vi "Close.vi"(8 "error in (no error)":errorcluster, 11 "State in":T1={"State"=enum."Idle", "Start Time"=timestamp(0 s since 1904-01-01), "Configuration"={"Cycle Period"=0.0, "Ismatech"={"VISA resource name"="", "Simulated?"=FALSE, "Pump Number"=1.0, "Reverse?"=FALSE}, "Masterflex"={"VISA resource name"="", "Simulated?"=FALSE, "Pump Number"=1.0, "Reverse?"=FALSE}, "Manual Entry"=0.0, "VICI Settings"={"VISA resource name"="", "Simulated?"=FALSE, "Pump Letter"="", "Reverse?"=FALSE}, "Output Device"=enum."Ismatec ISM 831C", "Tacmina Settings"={"Analog DAQ Task"="", "Digital DAQ Task"=""}, "KNF SIMDOS Settings"={"VISA resource name"="", "Simulated?"=TRUE}, "ASIA Pump C"={"ASIA Pump #"=0, "channel"=0, "Simulated"=FALSE}, "FLOM Settings"={"VISA resource name"="", "Simulated?"=TRUE, "Pump Number"=0.0}, "Pump Calibration File"=path "", "Calibration Slope"=0.0, "Calibration Y Intercept"=0.0, "Pump Cal Enum"=0, "SSI PR Settings"={"VISA resource name"="", "Simulated?"=FALSE}}, "Current Time"=timestamp(0 s since 1904-01-01), "First Iteration"=FALSE, "Data"={"Pump Speed"=0.0, "Pump Pressure"=0.0, "Pump Flow"=0.0}, "Process Name"="", "Pump On?"=enum."Off", "Output Error"=FALSE, "Log Started"=FALSE, "Overpressure Alarming"=FALSE} {"Configuration"."ASIA Pump C"."channel" min=0 max=1 step=1; "Configuration"."Masterflex"."Pump Number" min=1.0 max=20.0 step=1.0; "Configuration"."Ismatech"."Pump Number" min=1.0 max=20.0 step=1.0}) -> (0 "error out":errorcluster, 3 "State out":T1={"State"=enum."Idle", "Start Time"=timestamp(0 s since 1904-01-01), "Configuration"={"Cycle Period"=0.0, "Ismatech"={"VISA resource name"="", "Simulated?"=FALSE, "Pump Number"=1.0, "Reverse?"=FALSE}, "Masterflex"={"VISA resource name"="", "Simulated?"=FALSE, "Pump Number"=1.0, "Reverse?"=FALSE}, "Manual Entry"=0.0, "VICI Settings"={"VISA resource name"="", "Simulated?"=FALSE, "Pump Letter"="", "Reverse?"=FALSE}, "Output Device"=enum."Ismatec ISM 831C", "Tacmina Settings"={"Analog DAQ Task"="", "Digital DAQ Task"=""}, "KNF SIMDOS Settings"={"VISA resource name"="", "Simulated?"=TRUE}, "ASIA Pump C"={"ASIA Pump #"=0, "channel"=0, "Simulated"=FALSE}, "FLOM Settings"={"VISA resource name"="", "Simulated?"=TRUE, "Pump Number"=0.0}, "Pump Calibration File"=path "", "Calibration Slope"=0.0, "Calibration Y Intercept"=0.0, "Pump Cal Enum"=0, "SSI PR Settings"={"VISA resource name"="", "Simulated?"=FALSE}}, "Current Time"=timestamp(0 s since 1904-01-01), "First Iteration"=FALSE, "Data"={"Pump Speed"=0.0, "Pump Pressure"=0.0, "Pump Flow"=0.0}, "Process Name"="", "Pump On?"=enum."Off", "Output Error"=FALSE, "Log Started"=FALSE, "Overpressure Alarming"=FALSE} {"Configuration"."ASIA Pump C"."channel" min=0 max=1 step=1; "Configuration"."Masterflex"."Pump Number" min=1.0 max=20.0 step=1.0; "Configuration"."Ismatech"."Pump Number" min=1.0 max=20.0 step=1.0})   [LabVIEW 2018, in "Pump Module.lvlib" / "Pump Module Engine.lvlib"]
uses:
  Pump Module Engine.lvlib
  State Cluster.ctl
  State Enum.ctl
  Pump Module Settings Cluster.ctl
  Ismatec ISM 831C/Controls/Ismatech Settings Cluster.ctl
  Masterflex 7550-30/Controls/Settings Cluster.ctl
  VICI M50 Party Mode/Settings Cluster.ctl
  Measure Instrument/PID 2 Output Enum.ctl
  Tacmina QI/Tacmina QI DAQ Setting.ctl
  KNF Pump/Settings Cluster plus SIMDOS.ctl
  ASIA Pump/Pump Settings.ctl
  FLOM Pump/Settings Cluster.ctl
  SSI PR Class/SSI PR Settings Cluster.ctl
  Tag VIs/Tag FGV Operation Enum.ctl
  Masterflex 7550-30/Masterflex 7550-30.lvlib
  Ismatec ISM 831C/Ismatec ISM 831C.lvlib
  Tacmina QI/Tacmina QI.lvlib
  VICI M50 Party Mode/VICI M6 M50 Party Mode.lvlib
  ASIA Pump.lvlib
  KNF Pump/KNF SIMDOS.lvlib
  FLOM Pump/FLOM Pump.lvlib
  SSI PR Class/SSI PR Pump.lvlib
  Shared Variables/Dynamic Shared Variables.lvlib
  Pump Module.lvlib
panel:
  # "Output Instruments"
  # "Output Instruments"
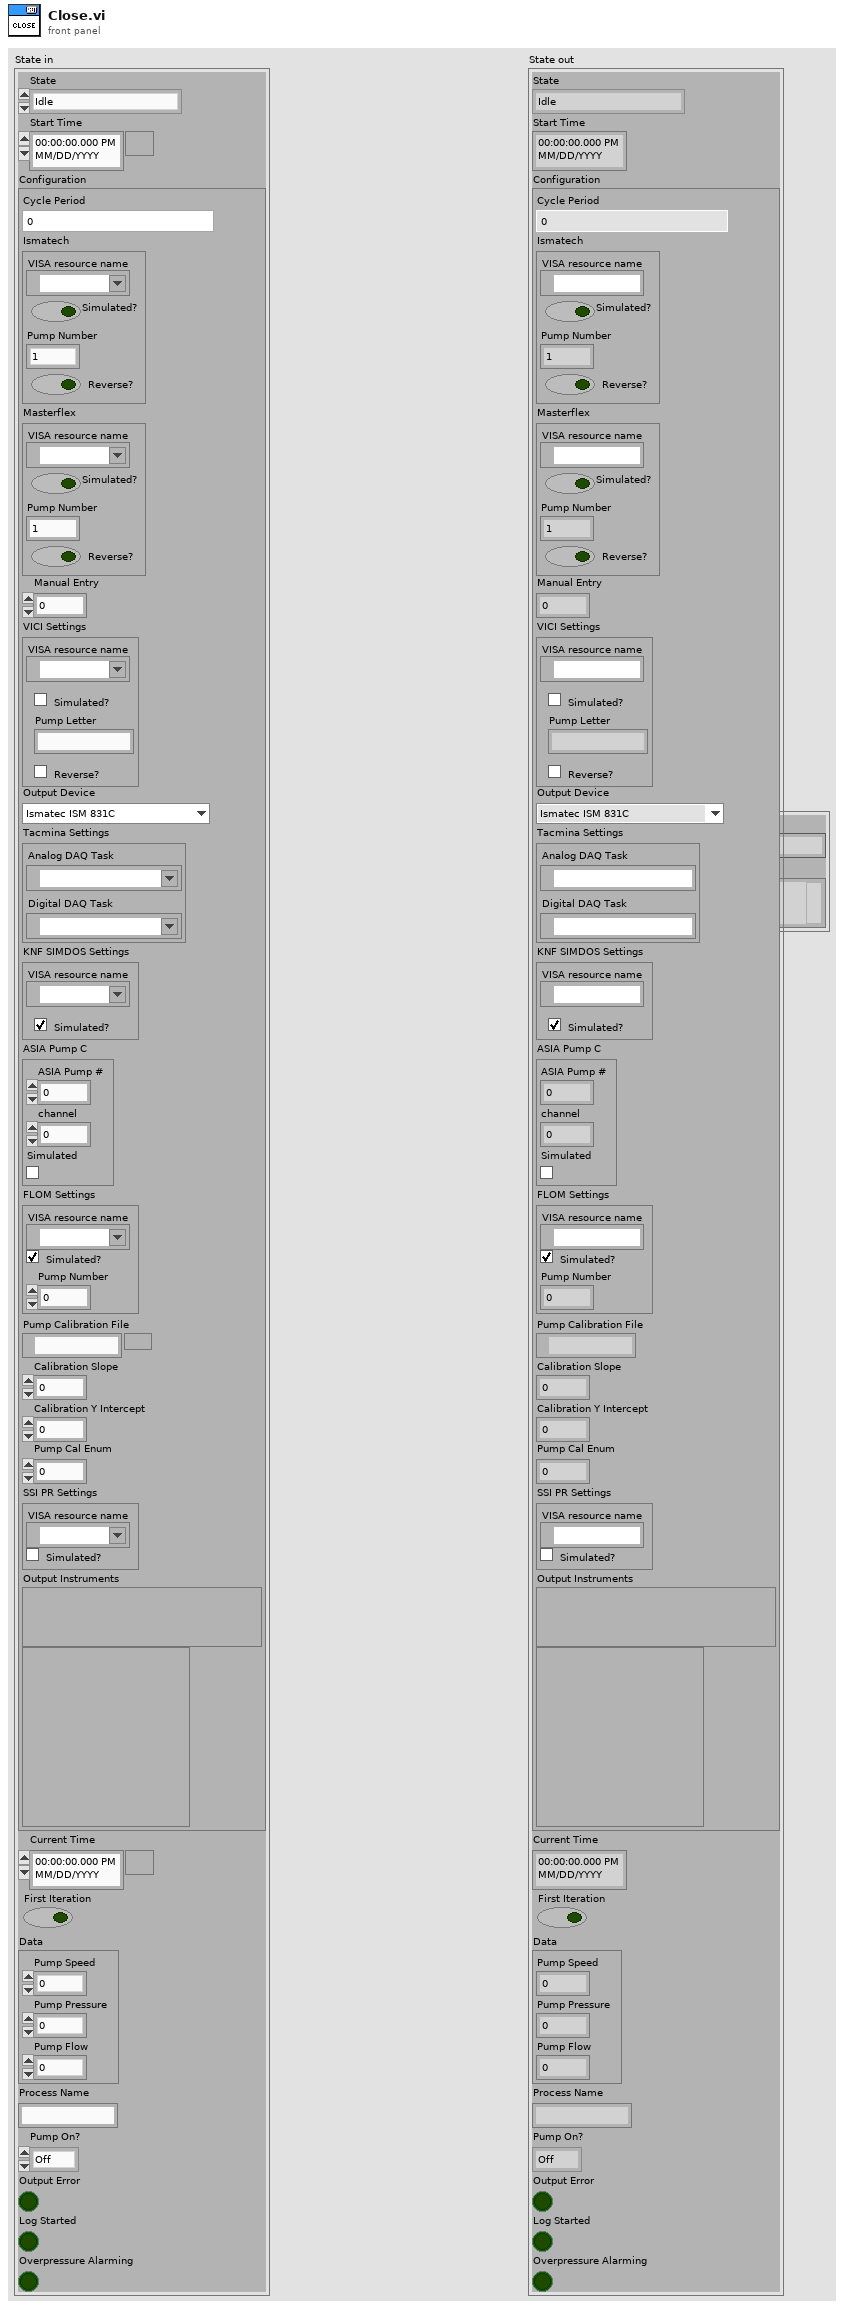
[diagram p1: front panel]
types:
  T1 = typedef "Pump Module.lvlib/Pump Module Engine.lvlib/State Cluster.ctl" = cluster{"State":T2, "Start Time":timestamp, "Configuration":T3, "Current Time":timestamp, "First Iteration":bool, "Data":cluster{"Pump Speed":dbl, "Pump Pressure":dbl, "Pump Flow":dbl}, "Process Name":string, "Pump On?":enum16{"Off", "On", "Not Initialized"}, "Output Error":bool, "Log Started":bool, "Overpressure Alarming":bool}
  T2 = typedef "Pump Module.lvlib/Pump Module Engine.lvlib/State Enum.ctl" = enum16{"Measuring", "Idle", "Paused"}
  T3 = typedef "Pump Module.lvlib/Pump Module Settings Cluster.ctl" = cluster{"Cycle Period":dbl, "Ismatech":T4, "Masterflex":T5, "Manual Entry":dbl, "VICI Settings":T6, "Output Device":T7, "Tacmina Settings":T8, "KNF SIMDOS Settings":T9, "ASIA Pump C":T10, "FLOM Settings":T11, "Pump Calibration File":path, "Calibration Slope":dbl, "Calibration Y Intercept":dbl, "Pump Cal Enum":u16, "SSI PR Settings":T12}
  T4 = typedef "Ismatec ISM 831C.lvlib/Ismatech Settings Cluster.ctl" = cluster{"VISA resource name":refnum<visa-resource-name>, "Simulated?":bool, "Pump Number":dbl, "Reverse?":bool}
  T5 = typedef "Masterflex 7550-30.lvlib/Settings Cluster.ctl" = cluster{"VISA resource name":refnum<visa-resource-name>, "Simulated?":bool, "Pump Number":dbl, "Reverse?":bool}
  T6 = typedef "VICI M6 M50 Party Mode.lvlib/Settings Cluster.ctl" = cluster{"VISA resource name":refnum<visa-resource-name>, "Simulated?":bool, "Pump Letter":string, "Reverse?":bool}
  T7 = typedef "PID 2 Output Enum.ctl" = enum16{"Default", "Ismatec ISM 831C", "Masterflex 7550-30", "VICI", "Tacmina QI", "KNF SIMDOS", "ASIA Type C", "FLOM UI-22-11", "SSI PR"}
  T8 = typedef "Tacmina QI.lvlib/Tacmina QI DAQ Setting.ctl" = cluster{"Analog DAQ Task":refnum<k21>, "Digital DAQ Task":refnum<k21>}
  T9 = typedef "KNF SIMDOS.lvlib/Settings Cluster plus SIMDOS.ctl" = cluster{"VISA resource name":refnum<visa-resource-name>, "Simulated?":bool}
  T10 = typedef "ASIA Pump.lvlib/Pump Settings.ctl" = cluster{"ASIA Pump #":i32, "channel":i32, "Simulated":bool}
  T11 = typedef "FLOM Pump.lvlib/Settings Cluster.ctl" = cluster{"VISA resource name":refnum<visa-resource-name>, "Simulated?":bool, "Pump Number":dbl}
  T12 = typedef "SSI PR Pump.lvlib/SSI PR Settings Cluster.ctl" = cluster{"VISA resource name":refnum<visa-resource-name>, "Simulated?":bool}
  T13 = typedef "Pump Module.lvlib/Pump Module Tag Names Cluster.ctl" = cluster{"Pump Speed":string, "Pump Flow":string, "Pump Pressure":string, "Output Device Tag":string, "Overpressure Tag":string}
  T14 = typedef "Tag FGV Operation Enum.ctl" = enum16{"Init", "Set Notification Queue", "Create Tag", "Commit", "Write Tag (Numeric)", "Write Tag (Boolean)", "Read All Tags", "Read One Tag", "Delete Tag Category", "Set Alarm Parameters (Numeric)", "Set Alarm Parameters (Boolean)", "Enable All Alarms", "Disable All Alarms", "Delete All Tags", "Read Alarms", "Ack Alarm", "Read Alarm Parameters (Numeric)", "Read Alarm Parameters (Boolean)"}
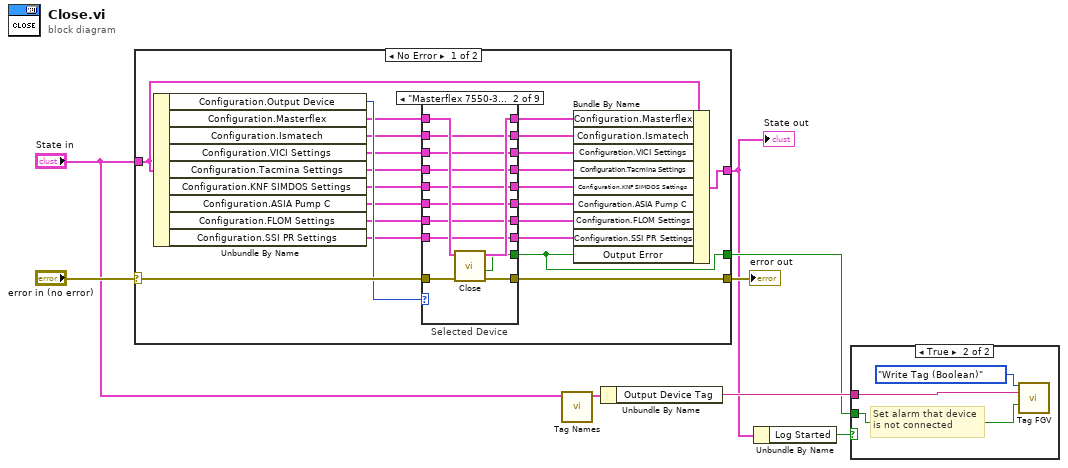
[diagram p0: block diagram]
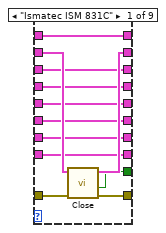
[diagram p3: hidden frame]
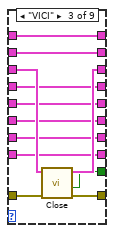
[diagram p4: hidden frame]
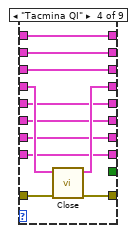
[diagram p5: hidden frame]
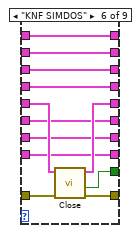
[diagram p7: hidden frame]
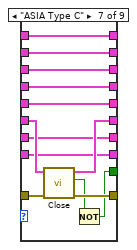
[diagram p8: hidden frame]
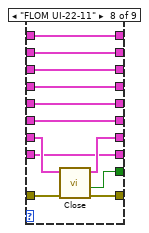
[diagram p9: hidden frame]
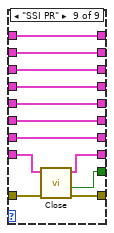
[diagram p10: hidden frame]
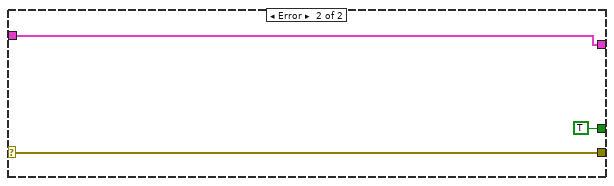
[diagram p11: hidden frame]
diagram:
  n1 = case shown="No Error" "error in (no error)" {
    selector: "error in (no error)" -> [w25 w138]
    tunnel: [w28 w138] -> w7
    tunnel: "State in" -> [w20 w137]
    tunnel: [w30 w137] -> w2
    tunnel: [w9 TRUE ("Connection Error")] -> w3
    frame No Error {
      n2 = Unbundle By Name(w20) -> ("Configuration.Output Device"=w19:T7, "Configuration.Masterflex"=w18:T5, "Configuration.Ismatech"=w17:T4, "Configuration.VICI Settings"=w16:T6, "Configuration.Tacmina Settings"=w15:T8, "Configuration.KNF SIMDOS Settings"=w14:T9, "Configuration.ASIA Pump C"=w13:T10, "Configuration.FLOM Settings"=w12:T11, "Configuration.SSI PR Settings"=w11:T12)
      n3 = case "Selected Device" shown="\"Masterflex 7550-30\"" w19 {
        tunnel: w18 -> [w38 w54 w61 w74 w86 w94 w109 w123 w135]
        tunnel: [w38 w53 w61 w74 w86 w94 w109 w123 w135] -> w29
        tunnel: w17 -> [w40 w51 w62 w75 w82 w93 w108 w122 w134]
        tunnel: [w42 w52 w64 w76 w85 w97 w110 w116 w127] -> w28
        tunnel: w25 -> [w41 w50 w65 w77 w85 w98 w111 w117 w128]
        tunnel: [w39 w51 w62 w75 w82 w93 w108 w122 w134] -> w27
        tunnel: w16 -> [w37 w49 w66 w72 w84 w92 w107 w121 w133]
        tunnel: [w37 w49 w63 w72 w84 w92 w107 w121 w133] -> w26
        tunnel: w15 -> [w36 w48 w60 w71 w83 w91 w106 w120 w132]
        tunnel: [w36 w48 w60 w73 w83 w91 w106 w120 w132] -> w24
        tunnel: w14 -> [w35 w47 w58 w70 w80 w96 w105 w119 w131]
        tunnel: [w35 w47 w58 w70 w80 w95 w105 w119 w131] -> w23
        tunnel: [w34 w46 w59 w69 w81 w90 w103 w118 w130] -> w22
        tunnel: w13 -> [w34 w46 w59 w69 w81 w90 w104 w118 w130]
        tunnel: w12 -> [w33 w45 w57 w68 w79 w89 w102 w115 w129]
        tunnel: [w33 w45 w57 w68 w79 w89 w102 w114 w129] -> w21
        tunnel: w11 -> [w32 w44 w56 w67 w78 w88 w101 w113 w126]
        tunnel: [w32 w44 w56 w67 w78 w88 w101 w113 w125] -> w10
        tunnel: [w31 w43 w55 _ _ w87 w99 w112 w124] -> w9
        frame "Ismatec ISM 831C" {
          n4 = call "Close.vi"("error in (no error)"=w41, "Ismatech Settings"=w40) -> ("error out"=w42:errorcluster, "Connection Error"=w31:bool, "Ismatech Settings"=w39:T4)  [unwired: 7 in]
        }
        frame "Masterflex 7550-30" {
          n5 = call "Close.vi"("error in (no error)"=w50, "Masterflex Settings in"=w54) -> ("error out"=w52:errorcluster, "Connection Error"=w43:bool, "Masterflex Settings out"=w53:T5)  [unwired: 7 in]
        }
        frame "VICI" {
          n6 = call "Close.vi"("error in (no error)"=w65, "VICI Settings"=w66) -> ("error out"=w64:errorcluster, "Connection Error"=w55:bool, "VICI Settings"=w63:T6)  [unwired: 7 in]
        }
        frame "Tacmina QI" {
          n7 = call "Close.vi"("error in"=w77, "Tacmina Settings in"=w71) -> ("error out"=w76:errorcluster, "Tacmina Settings out"=w73:T8)  [unwired: 8 in]
        }
        frame "Default", Default {
        }
        frame "KNF SIMDOS" {
          n8 = call "Close.vi"("error in (no error)"=w98, "KNF Settings"=w96) -> ("error out"=w97:errorcluster, "Connection Error"=w87:bool, "KNF Settings"=w95:T9)  [unwired: 7 in]
        }
        frame "ASIA Type C" {
          n9 = call "Close.vi"("error in (no error)"=w111, "ASIA Pump C"=w104) -> ("error out"=w110:errorcluster, "Task Completed"=w100:bool, "ASIA Pump C"=w103:T10)  [unwired: 7 in]
          n10 = Not(x=w100) -> (.not. x?=w99:bool)
        }
        frame "FLOM UI-22-11" {
          n11 = call "Close.vi"("error in (no error)"=w117, "FLOM Settings in"=w115) -> ("error out"=w116:errorcluster, "Connection Error"=w112:bool, "FLOM Settings out"=w114:T11)  [unwired: 7 in]
        }
        frame "SSI PR" {
          n12 = call "Close.vi"("error in (no error)"=w128, "SSI PR Settings In"=w126) -> ("error out"=w127:errorcluster, "Connection Error"=w124:bool, "SSI PR Settings Out"=w125:T12)  [unwired: 7 in]
        }
      }
      n13 = Bundle By Name(cluster=w20, "Configuration.Masterflex"=w29, "Configuration.Ismatech"=w27, "Configuration.VICI Settings"=w26, "Configuration.Tacmina Settings"=w24, "Configuration.KNF SIMDOS Settings"=w23, "Configuration.ASIA Pump C"=w22, "Configuration.FLOM Settings"=w21, "Configuration.SSI PR Settings"=w10, "Output Error"=w9) -> (w30:T1)
    }
    frame Error {
    }
  }
  "error out" <- w7
  "State out" <- w2
  n14 = call "Tag Names.vi"("State In"="State in") -> ("Pump Module Tag Names"=w5:T13)  [unwired: 8 in, 2 out]
  n15 = Unbundle By Name(w5) -> ("Output Device Tag"=w6:string)
  n16 = Unbundle By Name(w2) -> ("Log Started"=w1:bool)
  n17 = case shown="True" w1 {
    tunnel: w6 -> [_ w141]
    tunnel: w3 -> [_ w139]
    frame False {
    }
    frame True {
      # "Set alarm that device\nis not connected"
      n18 = call "Tag FGV.vi"("Operation"=Tag_FGV_Operation_Enum."Write Tag (Boolean)", "Tag Name"=w141, "Data"=w139) -> ()  [unwired: 5 in, 8 out]
    }
  }
